vi "AppMenuOptions.vi"(8 "error in (no error)":errorcluster, 10 "appMenu* in":refnum<k9>, 11 "FPGADMAChannelData in":refnum<class "FPGADMAChannelData.lvclass">) -> (0 "error out":errorcluster, 2 "appMenu* out":refnum<k9>, 3 "FPGADMAChannelData out":refnum<class "FPGADMAChannelData.lvclass">)   [LabVIEW 2013, in "FPGADMAChannelData.lvclass"]
uses:
  FPGADMAChannelData.lvclass
  xCE/xceRootNode/xceRootNode.lvclass
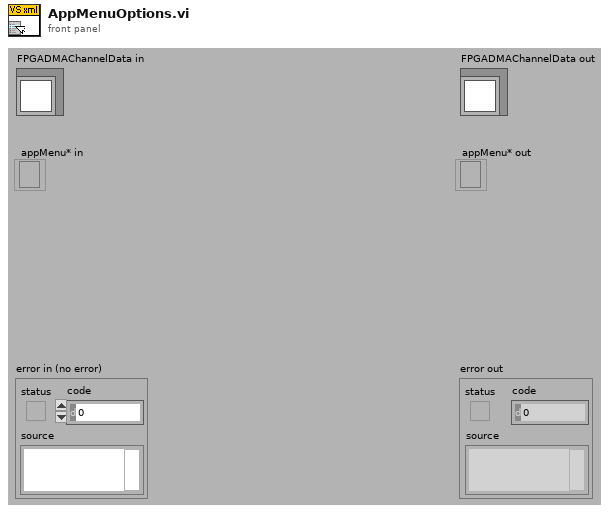
[diagram p1: front panel]
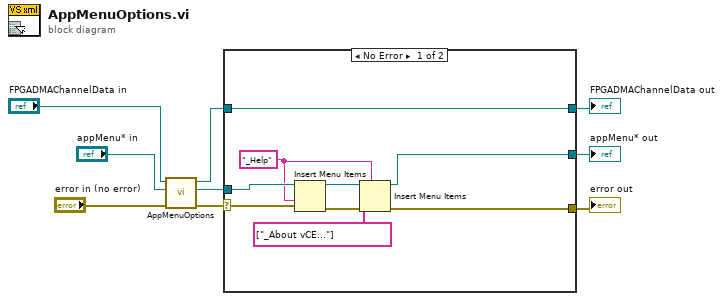
[diagram p0: block diagram]
diagram:
  n1 = call-parent "AppMenuOptions.vi"("error in (no error)"="error in (no error)", "appMenu* in"="appMenu* in", "xceRootNode in"="FPGADMAChannelData in") -> ("error out"=w6:errorcluster, "appMenu* out"=w5:refnum<k9>, "xceRootNode out"=w4:refnum<class "FPGADMAChannelData.lvclass">)  [unwired: 6 in]
  n2 = case shown="No Error" w6 {
    selector: w6 -> [w17 w21]
    tunnel: w5 -> [w16 w20]
    tunnel: w4 -> [w18 w19]
    tunnel: [w18 w19] -> w3
    tunnel: [w11 w20] -> w2
    tunnel: [w10 w21] -> w1
    frame No Error {
      w14 = "_Help"
      n3 = Insert Menu Items(6:w17, 7:w14, 9:w16) -> (0:w15:errorcluster, 3:w12:refnum<k9>)  [unwired: 3 in, 1 out]
      n4 = Insert Menu Items(5:w14, 6:w15, 7:string[] ["_About vCE..."] ("item tags"), 9:w12) -> (0:w10:errorcluster, 3:w11:refnum<k9>)  [unwired: 2 in, 1 out]
    }
    frame Error {
    }
  }
  "error out" <- w1
  "FPGADMAChannelData out" <- w3
  "appMenu* out" <- w2
